vi "Get Installed Test VI Path.vi"(8 "Error In":errorcluster, 9 "Files Installed":path[](array[path]), 10 "Test VI Path":path) -> (0 "Error Out":errorcluster, 1 "Found?":bool, 2 "Installed Test VI Path":path)   [LabVIEW 2014, in "LMH-Toolbox.lvlib" / "LMH-Installer Tools.lvlib"]
uses:
  <vilib>/MakerHub/Toolbox/Private/Installer Tools/LMH-Installer Tools.lvlib
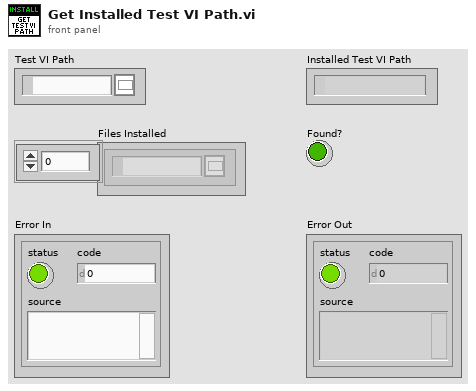
[diagram p1: front panel]
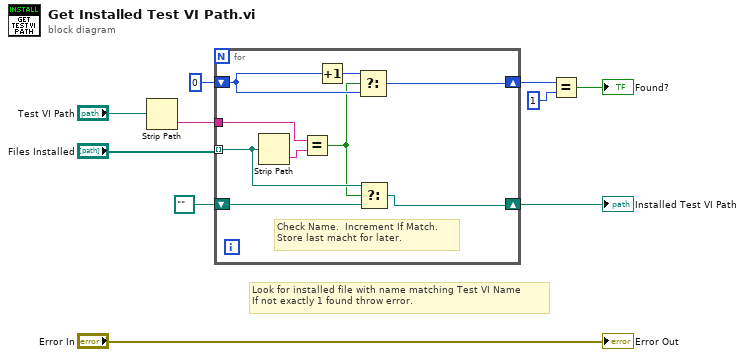
[diagram p0: block diagram]
diagram:
  # "Look for installed file with name matching Test VI Name\nIf not exactly 1 found throw error."
  n1 = Strip Path(path="Test VI Path") -> (name=w6:string)  [unwired: 1 out]
  n2 = for {
    tunnel: w6 -> [w19]
    shift-right: [w16] -> w3
    shift-left: 0 -> [w15]
    tunnel: "Files Installed" -> [w14] mode=indexing
    shift-right: [w11] -> w9
    shift-left: path "" -> [w12]
    # "Check Name.  Increment If Match.\nStore last macht for later."
    n3 = Strip Path(path=w14) -> (name=w18:string)  [unwired: 1 out]
    n4 = Equal?(x=w19, y=w18) -> (x = y?=w13:bool)
    n5 = Increment(x=w15) -> (x+1=w17:i32)
    n6 = Select(t=w17, s=w13, f=w15) -> (s? t:f=w16:i32)
    n7 = Select(t=w14, s=w13, f=w12) -> (s? t:f=w11:path)
  }
  "Installed Test VI Path" <- w9
  n8 = Equal?(x=w3, y=1) -> (x = y?=→"Found?":bool)
  "Error Out" <- "Error In"
